vi "SimpleHTTPServer.vi"(10 "Root Path (blank: ..\\html)":path) -> ()   [LabVIEW 2013]
uses:
  <vilib>/Utility/error.llb/DialogType.ctl
  <vilib>/Platform/browser.llb/Open URL in Default Browser (string).vi
panel:
  in  "Open Browser":bool
  in  "stop":bool
  in  "Port":u16=8000
  out "Requests":string[](array[string])
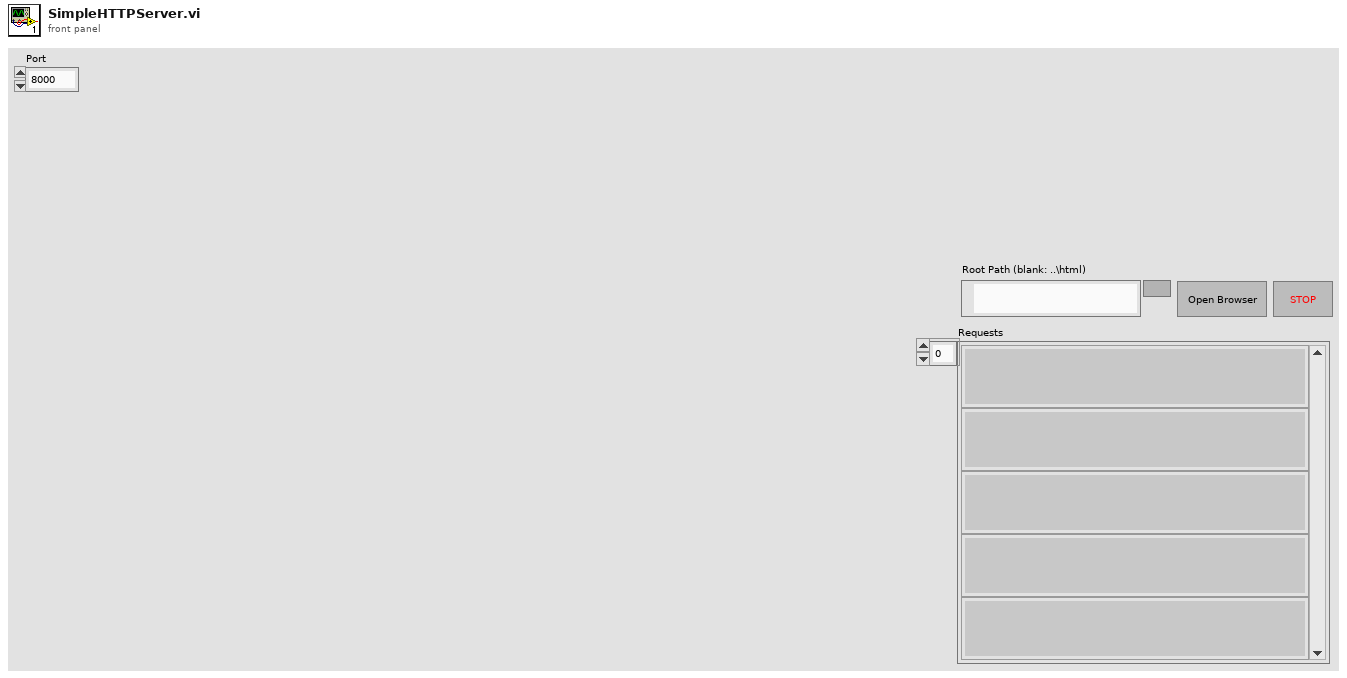
[diagram p1: front panel]
types:
  T1 = typedef "DialogType.ctl" = u16
  T2 = enum16{"Standard", "Buffered", "CRLF", "Immediate"}
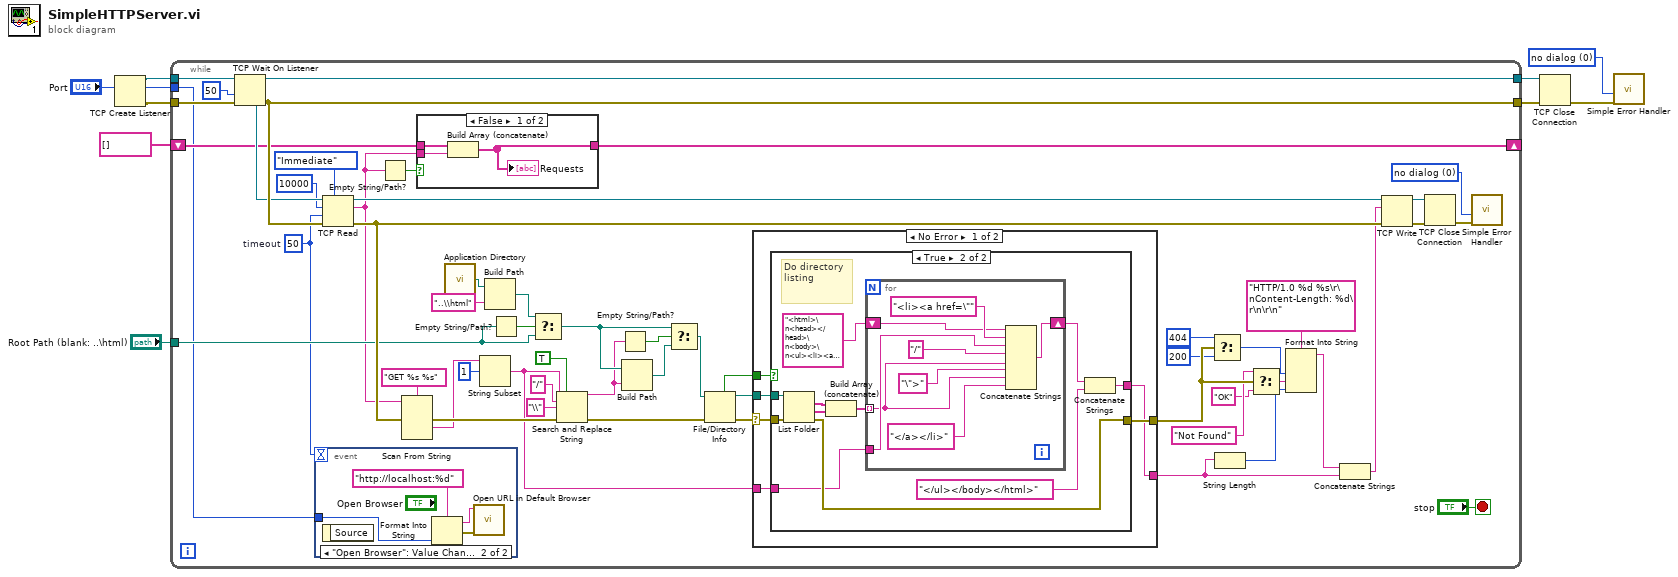
[diagram p0: block diagram]
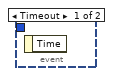
[diagram p2: hidden frame]
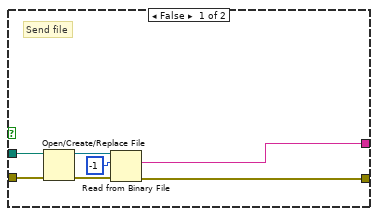
[diagram p4: hidden frame]
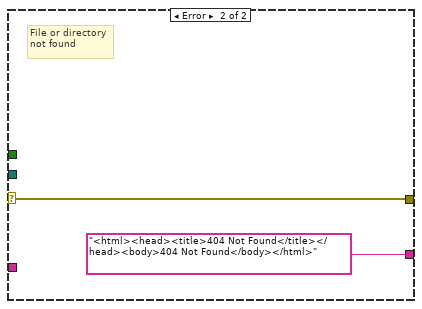
[diagram p5: hidden frame]
diagram:
  w2 = T1 0 items=["no dialog", "OK message", "continue or stop message", "OK message + warnings", "continue/stop + warnings"] ("type of dialog (OK msg:1)")
  n1 = TCP Create Listener(10:"Port") -> (0:w9:errorcluster, 2:w1:u16, 3:w8:refnum<k5>)  [unwired: 4 in]
  n2 = while {
    tunnel: "Root Path (blank: ..\\html)" -> [w27]
    tunnel: w9 -> [w24]
    tunnel: w8 -> [w23]
    tunnel: [w65] -> w7
    tunnel: [w22] -> w6
    shift-right: [w20] -> _
    shift-left: string[] [] ("Requests") -> [w21]
    tunnel: w1 -> [w11]
    stop <- "stop" stop-if-true
    w29 = T1 0 items=["no dialog", "OK message", "continue or stop message", "OK message + warnings", "continue/stop + warnings"] ("type of dialog (OK msg:1)")
    w12 = 50  # timeout
    n3 = TCP Wait On Listener(8:w24, 9:50 ("timeout ms (wait forever: -1)"), 11:w23) -> (0:w65:errorcluster, 3:w22:refnum<k5>, 4:w64:refnum<k5>)  [unwired: 1 in, 2 out]
    n4 = event shown="[1] \"Open Browser\": Value Change" {
      selector: _ -> [_ _]
      dyn-events: _ -> [_ _]
      timeout: w12 -> [_ _]
      tunnel: w11 -> [_ w66]
      event Timeout {
        n5 = event-data() -> ()  [unwired: 1 in, 1 out]
      }
      event "Open Browser": Value Change {
        n6 = event-data() -> ()  [unwired: 1 in, 1 out]
        n7 = Format Into String(format string="http://localhost:%d", w66) -> (resulting string=w69:string, error out=w68:errorcluster)  [unwired: 2 in]
        n8 = call-poly <vilib>:"Open URL in Default Browser.vi"("error in (no error)"=w68, "URL"=w69) -> ()  [unwired: 4 in, 2 out]
      }
    }
    n9 = TCP Read(connection ID=w64, bytes to read=10000, error in (no error)=w65, 7:T2."Immediate" ("mode (standard)"), 9:w12) -> (connection ID out=w42:refnum<k5>, data out=w15:string, error out=w62:errorcluster)
    n10 = Empty String/Path?(string/path=w15) -> (empty?=w16:bool)
    n11 = Scan From String(format string="GET %s %s", input string=w15, error in=w62) -> (error out=w60:errorcluster, output 1=w14:string)  [unwired: 4 in, 2 out]
    n12 = case shown="False" w16 {
      tunnel: w21 -> [w72 w73]
      tunnel: w15 -> [w71 _]
      tunnel: [w70 w73] -> w20
      frame False {
        n13 = Build Array (concatenate)(w72, w71) -> (w70:string[])
        "Requests" <- w70
      }
      frame True {
      }
    }
    n14 = call <vilib>:"Application Directory.vi"() -> ("Application Directory"=w18:path)
    n15 = String Subset(string=w14, offset (0)=1) -> (substring=w13:string)  [unwired: 1 in]
    n16 = Build Path(base path=w18, name or relative path="..\\html") -> (appended path=w17:path)
    n17 = Empty String/Path?(string/path=w27) -> (empty?=w55:bool)
    n18 = Select(t=w17, s=w55, f=w27) -> (s? t:f=w63:path)
    n19 = Search and Replace String(replace all?=TRUE ("replace all? (F)"), input string=w13, search string="/", replace string="\\" ("replace string (\"\")"), error in=w60) -> (result string=w50:string, error out=w30:errorcluster)  [unwired: 3 in, 2 out]
    n20 = Empty String/Path?(string/path=w50) -> (empty?=w49:bool)
    n21 = Build Path(base path=w63, name or relative path=w50) -> (appended path=w48:path)
    n22 = Select(t=w63, s=w49, f=w48) -> (s? t:f=w47:path)
    n23 = File/Directory Info(path=w47, error in=w30) -> (path out=w44:path, directory=w45:bool, error out=w46:errorcluster)  [unwired: 4 out]
    n24 = case shown="No Error" w46 {
      selector: w46 -> [w77 w107]
      tunnel: w45 -> [w79 _]
      tunnel: w44 -> [w78 _]
      tunnel: [w76 w107] -> w61
      tunnel: [w75 "<html><head><title>404 Not Found</title></head><body>404 Not Found</body></html>"] -> w32
      tunnel: w13 -> [w74 _]
      frame No Error {
        n25 = case shown="True" w79 {
          tunnel: w78 -> [w85 w96]
          tunnel: [w82 w92] -> w75
          tunnel: w77 -> [w81 w90]
          tunnel: [w80 w97] -> w76
          tunnel: w74 -> [_ w91]
          frame False {
            # "Send file"
            n26 = Open/Create/Replace File(file path (use dialog)=w85, error in=w81) -> (refnum out=w84:refnum<file>, error out=w86:errorcluster)  [unwired: 4 in, 1 out]
            n27 = Read from Binary File(8:w86, 10:-1 ("count (1)"), 11:w84) -> (0:w80:errorcluster, 2:w82:string)  [unwired: 3 in, 2 out]
          }
          frame True {
            # "Do directory listing"
            n28 = List Folder(path=w96, error in=w90) -> (filenames=w89:string[], folder names=w88:string[], error out=w97:errorcluster)  [unwired: 2 in, 1 out]
            n29 = Build Array (concatenate)(w89, w88) -> (w87:string[])
            n30 = for {
              shift-right: [w103] -> w94
              shift-left: "<html>\n<head></head>\n<body>\n<ul><li><a href=\"../\">../</a></li>" -> [w104]
              tunnel: w91 -> [w99]
              tunnel: w87 -> [w98] mode=indexing
              n31 = Concatenate Strings(w104, "<li><a href=\"", w99, "/" ("string"), w98, "\">", w98, "</a></li>" ("string")) -> (w103:string)
            }
            n32 = Concatenate Strings(w94, "</ul></body></html>") -> (w92:string)
          }
        }
      }
      frame Error {
        # "File or directory not found"
      }
    }
    n33 = Select(t=u16 404, s=w61, f=u16 200) -> (s? t:f=w36:u16)
    n34 = String Length(string=w32) -> (length=w35:i32)
    n35 = Select(t="Not Found", s=w61, f="OK") -> (s? t:f=w39:string)
    n36 = Format Into String(format string="HTTP/1.0 %d %s\r\nContent-Length: %d\r\n\r\n" ("data in"), w36, w39, w35) -> (resulting string=w59:string)  [unwired: 2 in, 1 out]
    n37 = Concatenate Strings(w59, w32) -> (w31:string)
    n38 = TCP Write(connection ID=w42, data in=w31, error in (no error)=w62) -> (connection ID out=w33:refnum<k5>, error out=w34:errorcluster)  [unwired: 1 in, 1 out]
    n39 = TCP Close Connection(connection ID=w33, error in (no error)=w34) -> (error out=w28:errorcluster)  [unwired: 1 in, 1 out]
    n40 = call <vilib>:"Simple Error Handler.vi"("type of dialog (OK msg:1)"=w29, "error in (no error)"=w28) -> ()  [unwired: 3 in, 5 out]
  }
  n41 = TCP Close Connection(connection ID=w6, error in (no error)=w7) -> (error out=w3:errorcluster)  [unwired: 1 in, 1 out]
  n42 = call <vilib>:"Simple Error Handler.vi"("type of dialog (OK msg:1)"=w2, "error in (no error)"=w3) -> ()  [unwired: 3 in, 5 out]
